vi "Set Trigger Mode.vi"(8 "error in (no error)":errorcluster, 10 "Trigger Mode":T1, 11 "DPO4104 in":refnum<class "DPO4104.lvclass">) -> (0 "error out":errorcluster, 3 "DPO4104 out":refnum<class "DPO4104.lvclass">)   [LabVIEW 2018, in "DPO4104.lvlib" / "DPO4104.lvclass"]
doc: "This Override sets the trigger to Auto or Normal mode. Auto generates a trigger even if one has not been detected after certain perios of time. Normal waits for trigger detection."
uses:
  DPO4104.lvclass
  PPLs/Oscilloscope/Parent/Oscilloscope.lvlibp/Custom Controls/Trigger Mode.ctl
  PPLs/Oscilloscope/Parent/Oscilloscope.lvlibp/Oscilloscope.lvclass
  <instrlib>/Tektronix DPO MSO 2000 4000 Series/Tektronix DPO MSO 2000 4000 Series.lvlib
  C:/Projects/LabVIEW/PPLs/Oscilloscope/Parent/Oscilloscope.lvlibp/Oscilloscope.lvclass
  PPLs/Oscilloscope/Parent/Oscilloscope.lvlibp
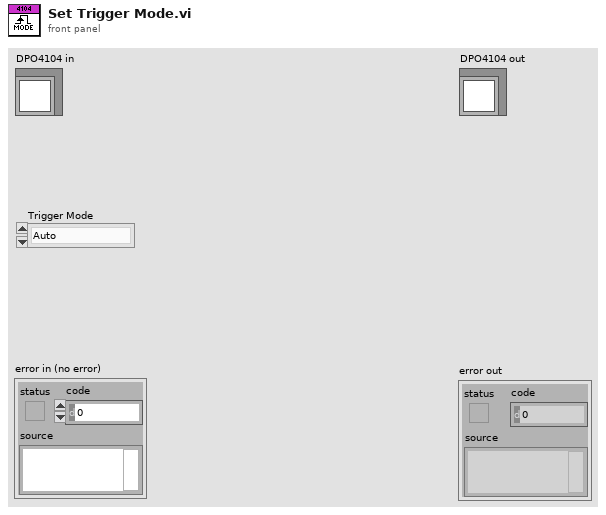
[diagram p1: front panel]
types:
  T1 = typedef "Oscilloscope.lvlibp/Trigger Mode.ctl" = enum16{"Auto", "Normal"}
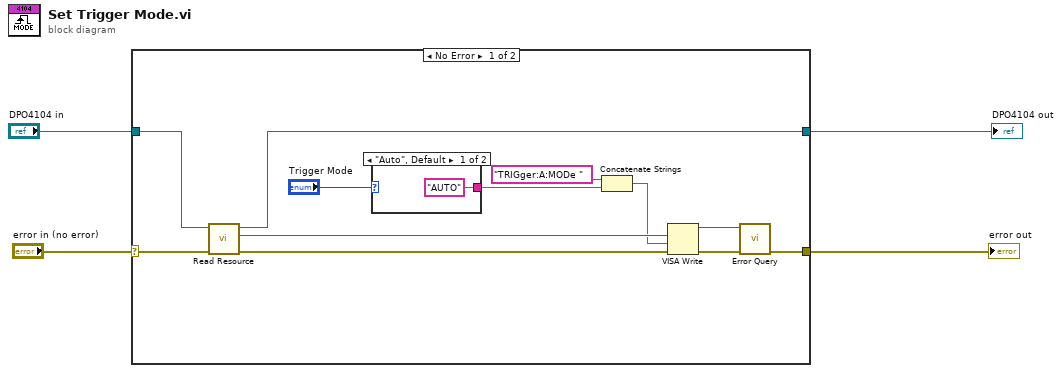
[diagram p0: block diagram]
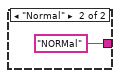
[diagram p2: hidden frame]
diagram:
  n1 = case shown="No Error" "error in (no error)" {
    selector: "error in (no error)" -> [w16 w20]
    tunnel: [w6 w20] -> w3
    tunnel: [w14 w19] -> w2
    tunnel: "DPO4104 in" -> [w15 w19]
    frame No Error {
      n2 = call "Read Resource.vi"("error in (no error)"=w16, "Oscilloscope in"=w15) -> ("error out"=w7:errorcluster, "Resource"=w8:refnum<visa-resource-name>, "Oscilloscope out"=w14:refnum<class "DPO4104.lvclass">)  [unwired: 7 in]
      n3 = case shown="\"Auto\", Default" "Trigger Mode" {
        tunnel: ["AUTO" "NORMal"] -> w11
        frame "Auto", Default {
        }
        frame "Normal" {
        }
      }
      n4 = Concatenate Strings("TRIGger:A:MODe " ("string"), w11) -> (w5:string)
      n5 = VISA Write(VISA resource name=w8, write buffer=w5, error in (no error)=w7) -> (VISA resource name out=w10:refnum<visa-resource-name>, error out=w9:errorcluster)  [unwired: 1 out]
      n6 = call <instrlib>:"Error Query.vi"("error in (no error)"=w9, "VISA resource name"=w10) -> ("error out"=w6:errorcluster)  [unwired: 6 in, 3 out]
    }
    frame Error {
    }
  }
  "error out" <- w3
  "DPO4104 out" <- w2
